vi "Kill Async Methods.vi"(8 "error in (no error)":errorcluster, 10 "VI Refnum":refnum<vi>) -> (0 "error out":errorcluster)   [LabVIEW 2021, in "Async Methods Actor.lvlib" / "Async Methods Actor.lvclass"]
uses:
  Async Methods Actor.lvclass
  <vilib>/ActorFramework/Actor/Actor.lvclass
  Async Methods Actor Messages/Async Message/Async Message.lvclass
  Async Methods Actor.lvclass/Async Methods Actor.ctl
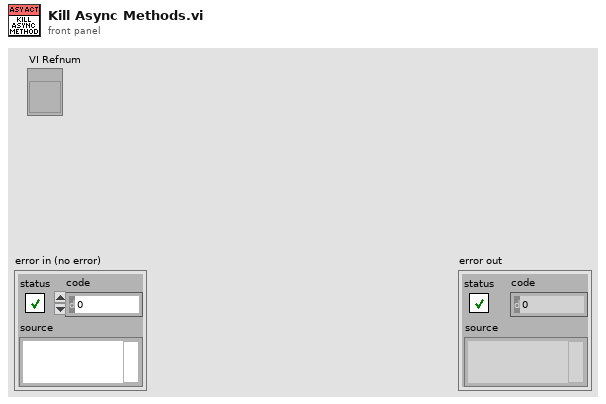
[diagram p1: front panel]
types:
  T1 = enum32{"Invalid", "Standard", "Closed", "Hidden", "Minimized", "Maximized"}
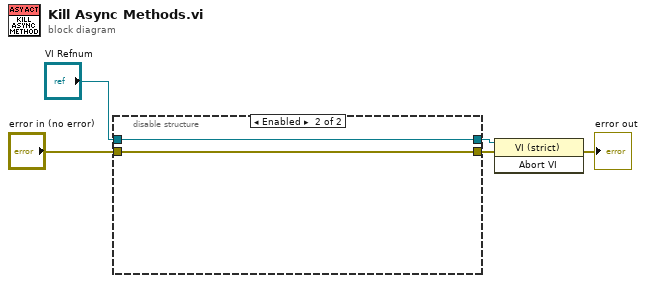
[diagram p0: block diagram]
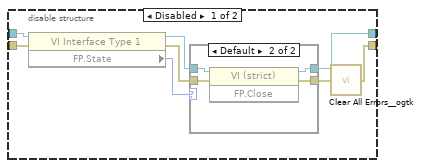
[diagram p2: hidden frame]
diagram:
  n1 = disable-structure shown="Enabled" {
    disable-tunnel: [w13 w21] -> w5
    disable-tunnel: [w11 w20] -> w3
    disable-tunnel: "error in (no error)" -> [w10 w20]
    disable-tunnel: "VI Refnum" -> [w6 w21]
    frame Disabled {
      n2 = property class="VI Interface Type 1"(reference=w6, error in=w10) -> (reference out=w7:refnum<vi>, error out=w9:errorcluster, "FP.State"=w8:T1)
      n3 = case shown="Default" w8 {
        tunnel: [w14 w19] -> w13
        tunnel: [w15 w18] -> w12
        tunnel: w9 -> [w15 w17]
        tunnel: w7 -> [w14 w16]
        frame "Invalid", "Closed" {
        }
        frame Default {
          n4 = invoke class="VI (strict)" method="FP.Close"(reference=w16, error in=w17) -> (reference out=w19:refnum<vi>, error out=w18:errorcluster)  [unwired: 1 in, 1 out]
        }
      }
      n5 = call <userlib>:"Clear All Errors__ogtk.vi"("Error In"=w12) -> ("Error Out"=w11:errorcluster)  [unwired: 3 in]
    }
    frame Enabled {
    }
  }
  n6 = invoke class="VI (strict)" method="Abort VI"(reference=w5, error in=w3) -> (error out=→"error out":errorcluster)  [unwired: 1 in, 2 out]
